vi "fpga_host.vi"() -> ()   [LabVIEW 2010]
uses:
  <vilib>/rvi/interface/nirviMethod/nirviMethod.xnode
  <vilib>/rvi/interface/nirviOpenFPGA/nirviOpenFPGA.xnode
  <vilib>/userDefined/High Color/nirio_resource_hc.ctl
  <vilib>/rvi/interface/nirviReadWriteControl/nirviReadWriteControl.xnode
  <vilib>/rvi/interface/nirviCloseFPGA/nirviCloseFPGA.xnode
  fpga_integrator.vi
  <vilib>/Analysis/NI_AALBase.lvlib
  <vilib>/rvi/errors/niLvFpgaWhatHappensToTopLevelVI.ctl
  <vilib>/rvi/interface/common/niFpgaNodeNameForErrorReporting.ctl
  <vilib>/rvi/errors/niLvFpgaAdjustHostInterfaceError.vi
  FPGA Bitfiles/ADC_test.lvproj_FPGA Target_fpga_integrator.vi.lvbitx
  <vilib>/RVI Host/nirviSupport.llb/nirviErrorClusterFromErrorCode.vi
  <vilib>/FPGAPlugInAG/PXI-7813R/niLvFpga_Close_PXI-7813R.vi
panel:
  in  "DIO34-1":bool
  in  "DIO32-1":bool
  in  "DIO34-0":bool
  in  "DIO32-0":bool
  out "channels graph":u32[][](graph)
  in  "Tab Control":T1(tab)=enum."channel 4"
  out "graph ch1":u32[](graph) caption="signal"
  out "hist ch1":T2(graph) caption="histogram"
  out "graph ch2":u32[](graph) caption="signal"
  out "hist ch2":T2(graph) caption="histogram"
  out "graph ch3":u32[](graph) caption="signal"
  out "hist ch3":T2(graph) caption="histogram"
  out "graph ch4":u32[](graph) caption="signal"
  out "hist ch4":T2(graph) caption="histogram"
  out "elements remaining in FIFO_DMA1":u32
  out "elements remaining in FIFO_DMA0":u32=284
  in  "read block size":u32=16000
  in  "number of pixels":i64=1000000000
  in  "iterations per pixel":i32=250
  in  "stop VI":bool
  in  "acquire?":bool
  # "ADC/FPGA integrator test program"
  # "Digital lines"
  # "© 2009 Helmchen group, Brain Research Institute, University of Zurich\n\nAuthors: \n- Dominik Langer, \n- Hansjörg Kasper, \n- Christoph Engelbrecht\n\nContact: helmchen@hifo.uzh.ch"
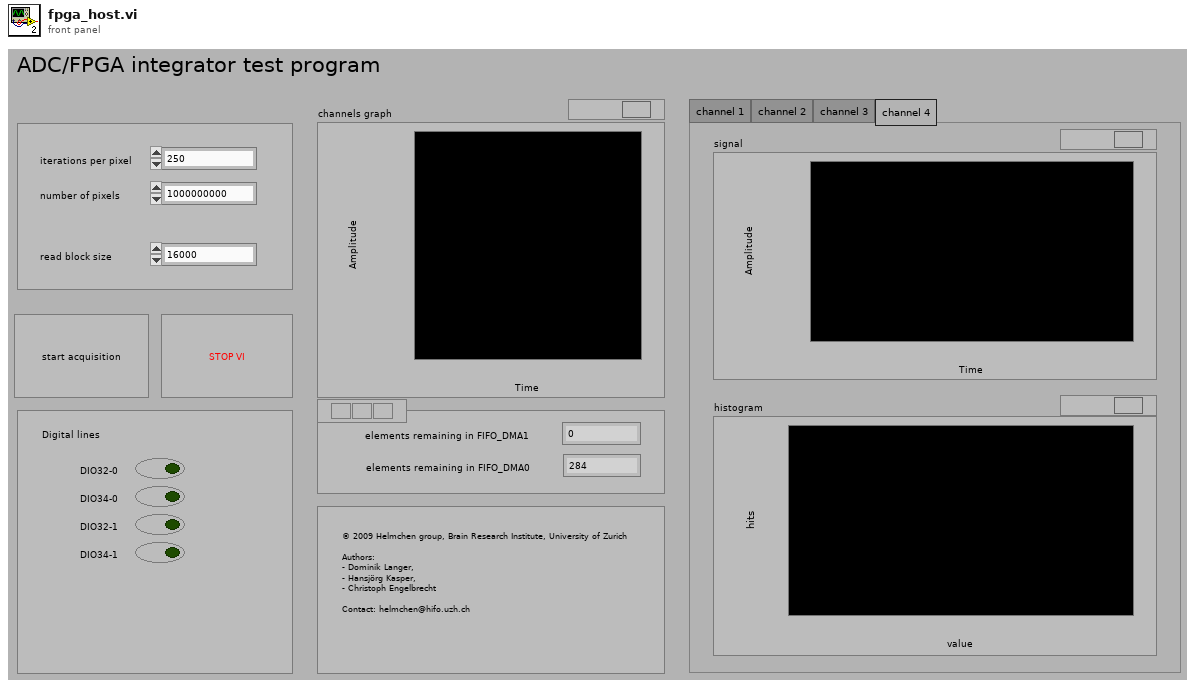
[diagram p1: front panel]
types:
  T1 = enum32{"channel 1", "channel 2", "channel 3", "channel 4"}
  T2 = cluster{"X Values":dbl[], "Histogram: h(x)":i32[]}
  T3 = typedef "nirio_resource_hc.ctl" = tag
  T4 = typedef "niFpgaNodeNameForErrorReporting.ctl" = enum16{"Open FPGA VI Reference", "Read/Write Control", "Invoke Method: Abort", "Invoke Method: Acknowledge IRQ", "Invoke Method: Download", "Invoke Method: FIFO.Configure", "Invoke Method: FIFO.Read", "Invoke Method: FIFO.Start", "Invoke Method: FIFO.Stop", "Invoke Method: FIFO.Write", "Invoke Method: Reset", "Invoke Method: Run", "Invoke Method: Wait on IRQ", "Close FPGA VI Reference"}
  T5 = typedef "niLvFpgaWhatHappensToTopLevelVI.ctl" = enum16{"top level VI scripted behind XNode", "top level VI inlined behind XNode"}
  T6 = cluster{"[0]":cluster{"X Values":dbl[], "Histogram: h(x)":i32[]}, "[1]":cluster{"X Values":dbl[], "Histogram: h(x)":i32[]}, "[2]":cluster{"X Values":dbl[], "Histogram: h(x)":i32[]}, "[3]":cluster{"X Values":dbl[], "Histogram: h(x)":i32[]}}
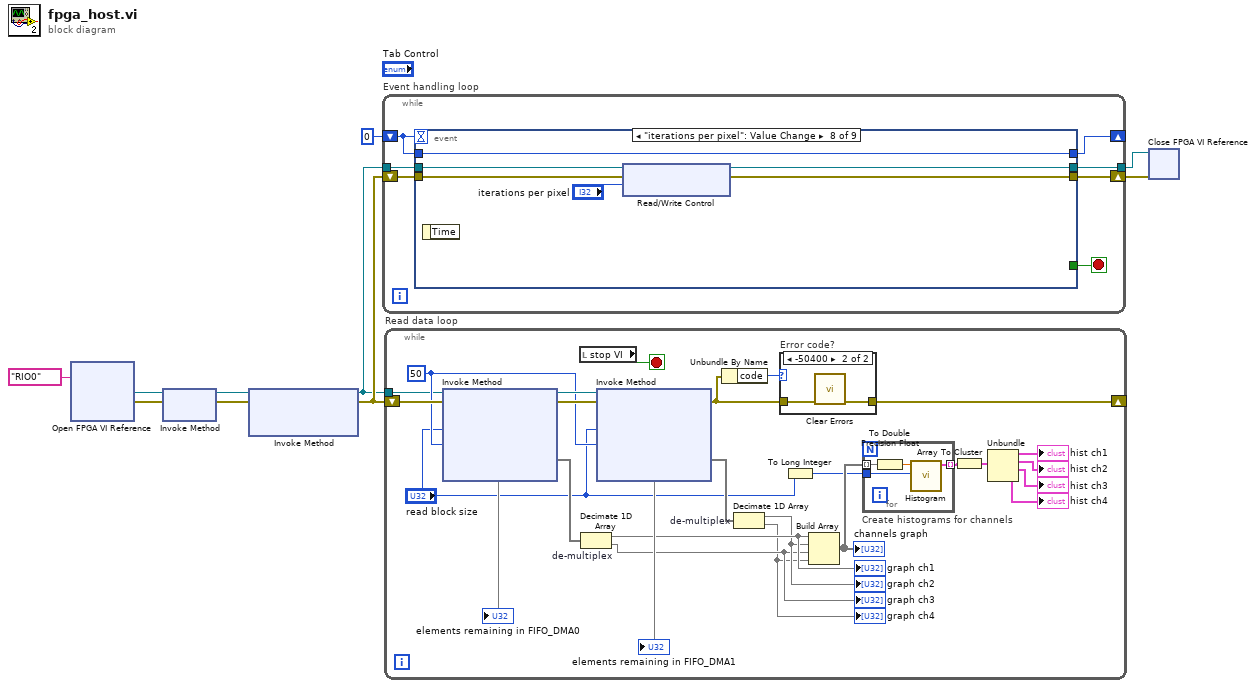
[diagram p0: block diagram]
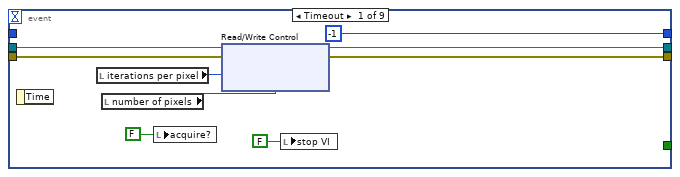
[diagram p2: hidden frame]
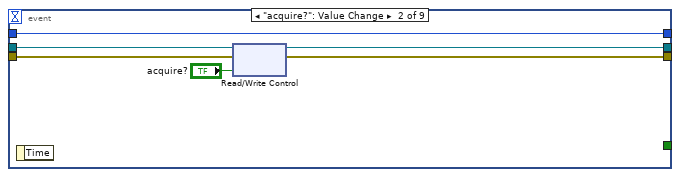
[diagram p3: hidden frame]
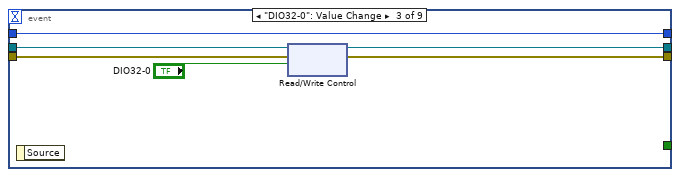
[diagram p4: hidden frame]
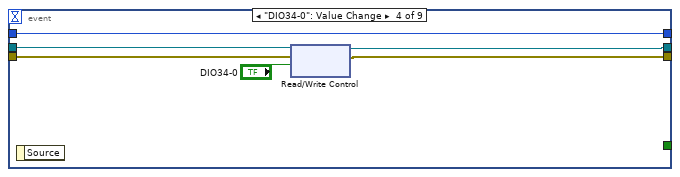
[diagram p5: hidden frame]
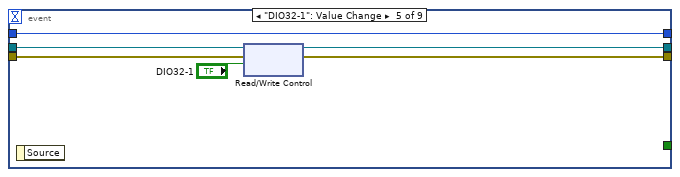
[diagram p6: hidden frame]
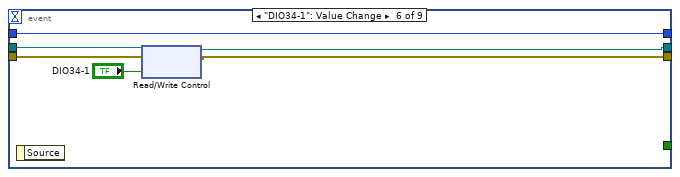
[diagram p7: hidden frame]
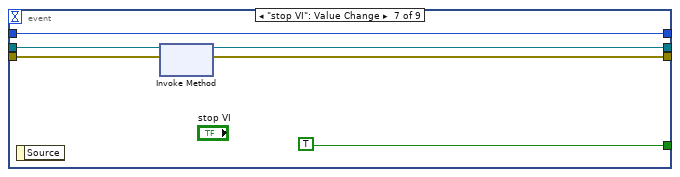
[diagram p8: hidden frame]
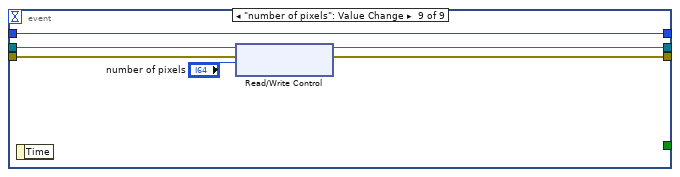
[diagram p9: hidden frame]
diagram:
  n1 = xnode "Open FPGA VI Reference"("resource name"=T3 "RIO0") -> ("FPGA VI Reference Out"=w3:refnum<k20>, "error out"=w4:errorcluster)  [unwired: 1 in]
  n2 = xnode "Invoke Method"("FPGA VI Reference In"=w3, "error in"=w4) -> ("FPGA VI Reference Out"=w5:refnum<k20>, "error out"=w6:errorcluster)
  n3 = xnode "Invoke Method"("FPGA VI Reference In"=w5, "error in"=w6) -> ("FPGA VI Reference Out"=w1:refnum<k20>, "error out"=w2:errorcluster)  [unwired: 1 out]
  n4 = while "Event handling loop" {
    shift-right: [w15] -> w9
    shift-left: w2 -> [w17]
    tunnel: w1 -> [w16]
    tunnel: [w14] -> w8
    shift-right: [w12] -> _
    shift-left: 0 -> [w11]
    stop <- w13 stop-if-true
    n5 = event shown="[7] \"iterations per pixel\": Value Change" {
      selector: _ -> [_ _ _ _ _ _ _ _ _]
      dyn-events: _ -> [_ _ _ _ _ _ _ _ _]
      timeout: w11 -> [_ _ _ _ _ _ _ _ _]
      tunnel: w17 -> [w25 w58 w85 w110 w139 w166 w192 w199 w224]
      tunnel: w16 -> [w24 w57 w83 w109 w138 w165 w189 w198 w223]
      tunnel: [w22 w56 w80 w107 w136 w162 w191 w196 w226] -> w15
      tunnel: [w23 w55 w82 w108 w135 w161 w190 w195 w225] -> w14
      tunnel: [_ _ _ _ _ _ TRUE _ _] -> w13
      tunnel: [-1 w53 w81 w112 w134 w163 w188 w194 w221] -> w12
      tunnel: w11 -> [_ w53 w81 w112 w134 w163 w188 w194 w221]
      event Timeout {
        n6 = event-data() -> ()  [unwired: 2 out]
        n7 = local read "iterations per pixel"() -> (w21:i32)
        n8 = local read "number of pixels"() -> (w20:i64)
        n9 = local write "acquire?"(FALSE ("acquire?")) -> ()
        n10 = xnode "Read/Write Control"("FPGA VI Reference In"=w24, "error in"=w25, "iterations per pixel"=w21, "number of pixels"=w20) -> ("FPGA VI Reference Out"=w23:refnum<k20>, "error out"=w22:errorcluster)
        n11 = local write "stop VI"(FALSE ("stop VI")) -> ()
      }
      event "acquire?": Value Change {
        n12 = event-data() -> ()  [unwired: 2 out]
        n13 = xnode "Read/Write Control"("FPGA VI Reference In"=w57, "error in"=w58, "acquire"="acquire?") -> ("FPGA VI Reference Out"=w55:refnum<k20>, "error out"=w56:errorcluster)
      }
      event "DIO32-0": Value Change {
        n14 = event-data() -> ()  [unwired: 2 out]
        n15 = xnode "Read/Write Control"("FPGA VI Reference In"=w83, "error in"=w85, "DIO32-0"="DIO32-0") -> ("FPGA VI Reference Out"=w82:refnum<k20>, "error out"=w80:errorcluster)
      }
      event "DIO34-0": Value Change {
        n16 = event-data() -> ()  [unwired: 2 out]
        n17 = xnode "Read/Write Control"("FPGA VI Reference In"=w109, "error in"=w110, "DIO34-0"="DIO34-0") -> ("FPGA VI Reference Out"=w108:refnum<k20>, "error out"=w107:errorcluster)
      }
      event "DIO32-1": Value Change {
        n18 = event-data() -> ()  [unwired: 2 out]
        n19 = xnode "Read/Write Control"("FPGA VI Reference In"=w138, "error in"=w139, "DIO32-1"="DIO32-1") -> ("FPGA VI Reference Out"=w135:refnum<k20>, "error out"=w136:errorcluster)
      }
      event "DIO34-1": Value Change {
        n20 = event-data() -> ()  [unwired: 2 out]
        n21 = xnode "Read/Write Control"("FPGA VI Reference In"=w165, "error in"=w166, "DIO34-1"="DIO34-1") -> ("FPGA VI Reference Out"=w161:refnum<k20>, "error out"=w162:errorcluster)
      }
      event "stop VI": Value Change {
        n22 = event-data() -> ()  [unwired: 2 out]
        n23 = xnode "Invoke Method"("FPGA VI Reference In"=w189, "error in"=w192) -> ("FPGA VI Reference Out"=w190:refnum<k20>, "error out"=w191:errorcluster)
      }
      event "iterations per pixel": Value Change {
        n24 = event-data() -> ()  [unwired: 2 out]
        n25 = xnode "Read/Write Control"("FPGA VI Reference In"=w198, "error in"=w199, "iterations per pixel"="iterations per pixel") -> ("FPGA VI Reference Out"=w195:refnum<k20>, "error out"=w196:errorcluster)
      }
      event "number of pixels": Value Change {
        n26 = event-data() -> ()  [unwired: 2 out]
        n27 = xnode "Read/Write Control"("FPGA VI Reference In"=w223, "error in"=w224, "number of pixels"="number of pixels") -> ("FPGA VI Reference Out"=w225:refnum<k20>, "error out"=w226:errorcluster)
      }
    }
  }
  n28 = while "Read data loop" {
    tunnel: w1 -> [w264]
    shift-right: [w249] -> _
    shift-left: w2 -> [w273]
    stop <- w268 stop-if-true
    w267 = 50 ("Timeout (ms)")
    n29 = xnode "Invoke Method"("FPGA VI Reference In"=w264, "error in"=w273, "Number of Elements"="read block size", "Timeout (ms)"=w267) -> ("FPGA VI Reference Out"=w271:refnum<k20>, "error out"=w272:errorcluster, "Data"=w270:void[], "Elements Remaining"=→"elements remaining in FIFO_DMA0")
    n30 = local read "stop VI"() -> (w268:bool)
    n31 = Decimate 1D Array "de-multiplex"(w270) -> (w259:void[], w257:void[])
    "graph ch3" <- w257
    "graph ch1" <- w259
    n32 = xnode "Invoke Method"("FPGA VI Reference In"=w271, "error in"=w272, "Number of Elements"="read block size", "Timeout (ms)"=w267) -> ("error out"=w265:errorcluster, "Data"=w269:void[], "Elements Remaining"=→"elements remaining in FIFO_DMA1")  [unwired: 1 out]
    n33 = Unbundle By Name(w265) -> ("code"=w266:i32)
    n34 = Decimate 1D Array "de-multiplex"(w269) -> (w258:void[], w256:void[])
    "graph ch2" <- w258
    "graph ch4" <- w256
    n35 = case "Error code?" shown="-50400" w266 {
      tunnel: w265 -> [w278 w280]
      tunnel: [w278 w279] -> w249
      frame 0, Default {
      }
      frame -50400 {
        n36 = call <vilib>:"Clear Errors.vi"("error in (no error)"=w280) -> ("error out"=w279:errorcluster)  [unwired: 6 out]
      }
    }
    n37 = To Long Integer(number="read block size") -> (32bit integer=w260:i32)
    n38 = Build Array(w259, w258, w257, w256) -> (w261:void[])
    "channels graph" <- w261
    n39 = for "Create histograms for channels" {
      tunnel: w261 -> [w277] mode=indexing
      tunnel: w260 -> [w275]
      tunnel: [w274] -> w255 mode=indexing
      n40 = To Double Precision Float(number=w277) -> (double precision float=w276:dbl)
      n41 = call <vilib>:"Histogram.vi"("intervals"=w275, "X"=w276) -> ("Histogram Graph"=w274:T2)  [unwired: 9 out]
    }
    n42 = Array To Cluster(array=w255) -> (cluster=w254:T6)
    n43 = Unbundle(w254) -> ("[0]"=→"hist ch1":T2, "[1]"=→"hist ch2":T2, "[2]"=→"hist ch3":T2, "[3]"=→"hist ch4":T2)
  }
  n44 = xnode "Close FPGA VI Reference"("FPGA VI Reference In"=w8, "error in"=w9) -> ()  [unwired: 1 out]
